vi "CovarianceToCorrelation.vi"(1 "covariance matrix":T1) -> (0 "Correlation table":string[][](array[string]))   [LabVIEW 2016]
uses:
  <vilib>/Analysis/Matrix/Datatypes/RealMatrix.ctl
  <vilib>/Analysis/Matrix/NI_Matrix.lvlib
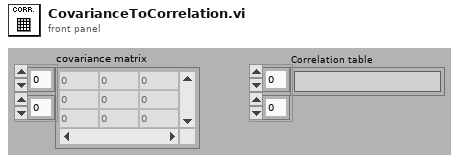
[diagram p1: front panel]
types:
  T1 = typedef "NI_Matrix.lvlib/RealMatrix.ctl" = dbl[][]
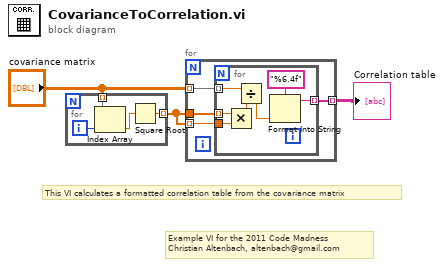
[diagram p0: block diagram]
diagram:
  # "Example VI for the 2011 Code Madness\nChristian Altenbach, altenbach@gmail.com"
  # "This VI calculates a formatted correlation table from the covariance matrix"
  n1 = for {
    tunnel: "covariance matrix" -> [w6] mode=indexing
    tunnel: [w4] -> w2 mode=indexing
    i -> [w7]
    n2 = Index Array(array=w6, index=w7) -> (element=w5:dbl)
    n3 = Square Root(x=w5) -> (sqrt(x)=w4:dbl)
  }
  n4 = for {
    tunnel: "covariance matrix" -> [w11] mode=indexing
    tunnel: w2 -> [w10]
    tunnel: w2 -> [w9] mode=indexing
    tunnel: [w8] -> w1 mode=indexing
    n5 = for {
      tunnel: w11 -> [w16] mode=indexing
      tunnel: w10 -> [w18] mode=indexing
      tunnel: w9 -> [w17]
      tunnel: [w12] -> w8 mode=indexing
      n6 = Multiply(x=w18, y=w17) -> (x*y=w15:dbl)
      n7 = Divide(x=w16, y=w15) -> (x/y=w14:dbl)
      n8 = Format Into String(format string="%6.4f", w14) -> (resulting string=w12:string)  [unwired: 2 in, 1 out]
    }
  }
  "Correlation table" <- w1
